vi "set_is_color.vi"(8 "error in (no error)":errorcluster, 10 "color?":bool, 11 "ColorOverlay in":refnum<class "ColorOverlay.lvclass">) -> (0 "error out":errorcluster, 3 "ColorOverlay out":refnum<class "ColorOverlay.lvclass">)   [LabVIEW 2010, in "ColorOverlay.lvclass"]
uses:
  ColorOverlay.lvclass
  ColorOverlay.lvclass/ColorOverlay.ctl
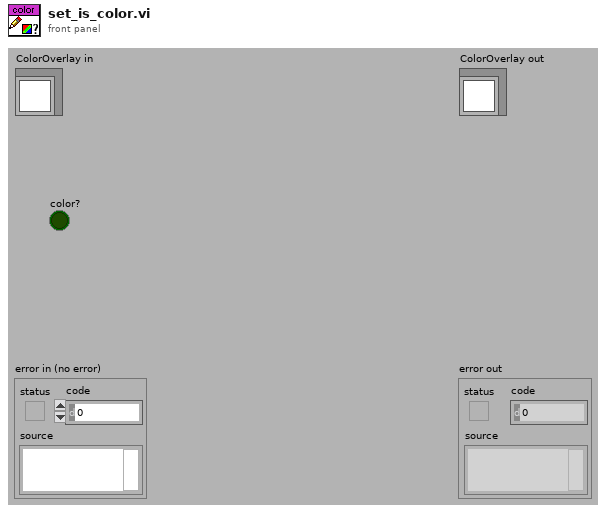
[diagram p1: front panel]
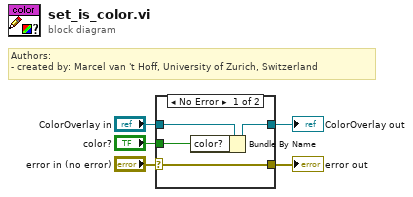
[diagram p0: block diagram]
diagram:
  # "Authors: \n- created by: Marcel van 't Hoff, University of Zurich, Switzerland"
  n1 = case shown="No Error" "error in (no error)" {
    selector: "error in (no error)" -> [w9 w11]
    tunnel: [w9 w11] -> w4
    tunnel: [w7 w10] -> w2
    tunnel: "ColorOverlay in" -> [w8 w10]
    tunnel: "color?" -> [w6 _]
    frame No Error {
      n2 = Bundle By Name(cluster=w8, "color?"=w6) -> (w7:refnum<class "ColorOverlay.lvclass">)
    }
    frame Error {
    }
  }
  "error out" <- w4
  "ColorOverlay out" <- w2
